vi "action.vi"(0 "HGF_TaskDFSM":refnum<class "HGF_TaskDFSM.lvclass">, 5 "error in (no error)":errorcluster, 8 "HGF_ThreadWorker":refnum<class "HGF_ThreadWorker.lvclass">) -> (10 "dup HGF_ThreadWorker":refnum<class "HGF_ThreadWorker.lvclass">, 14 "dup HGF_TaskDFSM":refnum<class "HGF_TaskDFSM.lvclass">, 19 "error out":errorcluster)   [LabVIEW 2012, in "HGF_DeviceFSM.lvlib" / "HGF_TaskDFSM.lvclass"]
uses:
  HGF_TaskDFSM.lvclass
  HGF_DeviceBaseClasses/HGF_DeviceVisitor/HGF_DeviceVisitor.lvclass
  HGF_DeviceFSM/HGF_DeviceFSM.lvsc/Trigger.ctl
  HGF_DeviceFSM/HGF_DeviceFSM.lvsc
  <vilib>/Statechart/Nodes/EventFiring/NI_SC_EventFiringNode.xnode
  HGF_DeviceFSM/HGF_DeviceFSM.lvsc/Inputs.ctl
  HGF_DeviceFSM/HGF_DeviceFSM.lvsc/Outputs.ctl
  HGF_DeviceFSM/HGF_DeviceFSM.lvsc/State.ctl
  HGF_DeviceFSM/HGF_DeviceFSM.lvsc/StatechartState.ctl
  <vilib>/Statechart/Infrastructure/RTStatechart/RunTime SCN.xnode
  HGF_BaseClasses/HGF_ThreadTask/HGF_ThreadTask.lvclass
  HGF_BaseClasses/HGF_Stop/HGF_Stop.lvclass
  HGF_BaseClasses/HGF_Exception/HGF_Exception.lvclass
  HGF_BaseClasses/HGF_Visitor/HGF_Visitor.lvclass
  HGF_BaseClasses/HGF_Event/HGF_Event.lvclass
  HGF_BaseClasses/HGF_TriggeredEvent/HGF_TriggeredEvent.lvclass
  HGF_BaseClasses/HGF_PVPublisher/HGF_PVPublisher.lvclass
  HGF_DFSMVisitor/HGF_DFSMVisitor.lvclass
  HGF_BaseClasses/HGF_Factory/HGF_Factory.lvclass
  HGF_BaseClasses/HGF_VariantDataObject/HGF_VariantDataObject.lvclass
  HGF_DeviceFSM/HGF_DeviceFSM_Internals.ctl
  HGF_DeviceBaseClasses/HGF_DeviceBaseClasses.lvlib
  <vilib>/Statechart/Common/IntGuid.ctl
  <vilib>/Statechart/Common/NI_SC_LVSCCommonFiles.lvlib
  HGF_DeviceFSM/HGF_DeviceFSM.lvsc/CompanionDiagram.vi/28/SC Main.vi
  <vilib>/Statechart/Common/DbgID.ctl
  HGF_BaseClasses/HGF_ThreadWorker/HGF_ThreadWorker.lvclass
panel:
  out "className":string
  out "Active States":T1
  out "DFSM Internals":T3
  out "SC Loop":i32
  out "Trigger timed out?":bool
  in  "Inputs":T4
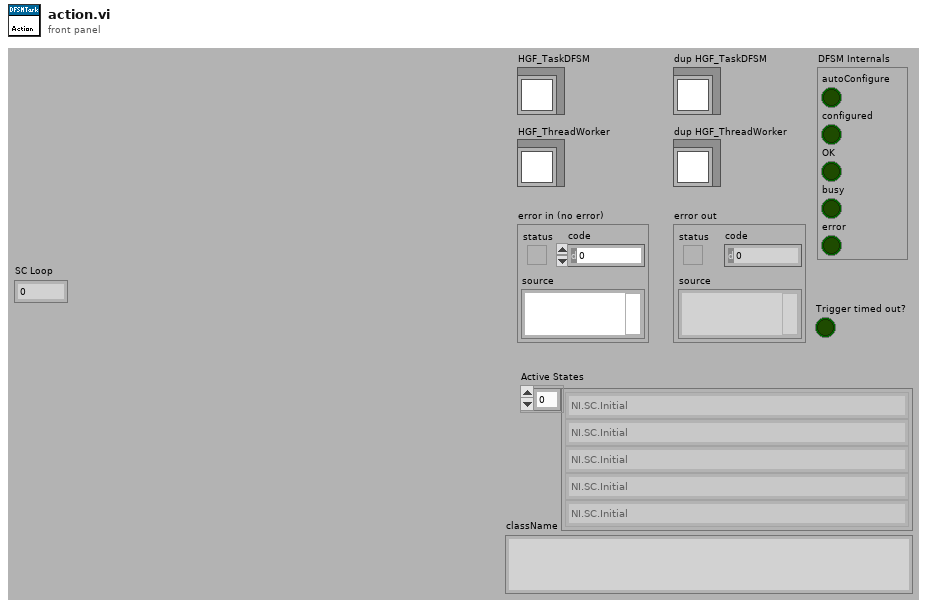
[diagram p1: front panel]
types:
  T1 = typedef "HGF_DeviceFSM.lvlib/HGF_DeviceFSM.lvsc/StatechartState.ctl" = T2[]
  T2 = typedef "HGF_DeviceFSM.lvlib/HGF_DeviceFSM.lvsc/State.ctl" = enum16{"NI.SC.Initial", "NI.SC.History", "NI.SC.ShallowHistory", "NI.SC.Terminal", "Alive", "Alive\\LiveCycle\\Configure", "Alive\\LiveCycle\\Configured", "Alive\\LiveCycle\\Error", "Alive\\LiveCycle\\NotConfigured", "Alive\\LiveCycle\\Configured\\ConfiguredRegion\\Busy", "Alive\\LiveCycle\\Configured\\ConfiguredRegion\\Idle", "Alive\\LiveCycle\\Configured\\ConfiguredRegion\\Idle\\IdleRegion\\Fault", "Alive\\LiveCycle\\Configured\\ConfiguredRegion\\Idle\\IdleRegion\\OK"}
  T3 = typedef "HGF_DeviceBaseClasses.lvlib/HGF_DeviceFSM_Internals.ctl" = cluster{"autoConfigure":bool, "configured":bool, "OK":bool, "busy":bool, "error":bool}
  T4 = typedef "HGF_DeviceFSM.lvlib/HGF_DeviceFSM.lvsc/Inputs.ctl" = cluster{"HGF_DeviceVisitor":refnum<class "HGF_DeviceVisitor.lvclass">, "autoConfigure":bool, "HGF_Factory":refnum<class "HGF_Factory.lvclass">, "DeviceInitData":refnum<class "HGF_VariantDataObject.lvclass">}
  T5 = typedef "HGF_DeviceFSM.lvlib/HGF_DeviceFSM.lvsc/Trigger.ctl" = enum16{"NULL", "configure", "fault", "error", "resetError", "STOP", "visit", "not_configured", "done", "ok", "previsit", "configured"}
  T6 = typedef "NI_SC_LVSCCommonFiles.lvlib/IntGuid.ctl" = cluster{"Data1":u32, "Data2":u16, "Data3":u16, "Data4":u8, "Data5":u8, "Data6":u8, "Data11":u8, "Data9":u8, "Data10":u8, "Data8":u8, "Data7":u8}
  T7 = typedef "NI_SC_LVSCCommonFiles.lvlib/DbgID.ctl" = cluster{"VIRef":u32, "IntGUID":T6}
  T8 = typedef "HGF_DeviceFSM.lvlib/HGF_DeviceFSM.lvsc/Outputs.ctl" = cluster{"HGF_DeviceVisitor":refnum<class "HGF_DeviceVisitor.lvclass">, "DFSM Internals":T3, "error out":errorcluster}
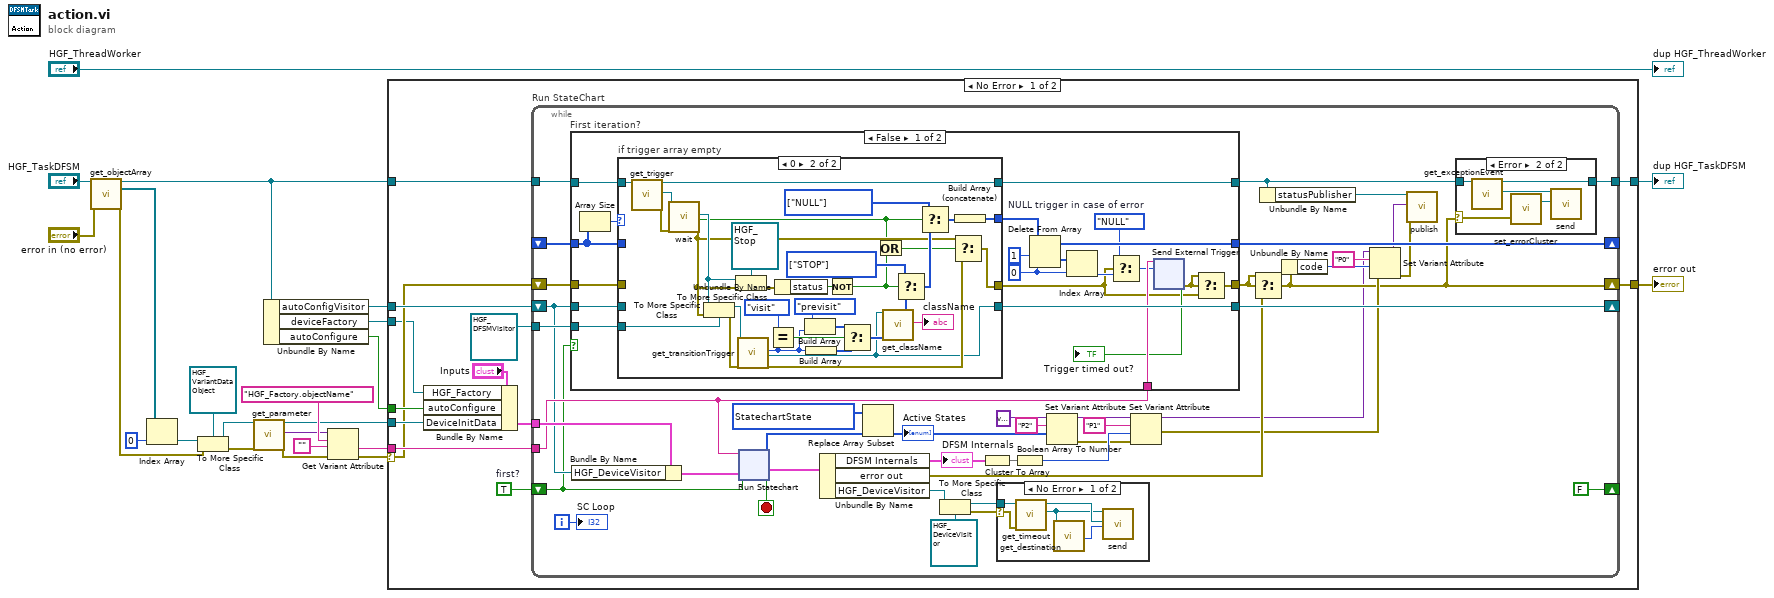
[diagram p0: block diagram]
diagram:
  n1 = call "get_objectArray.vi"("HGF_ThreadTask"="HGF_TaskDFSM", "error in (no error)"="error in (no error)") -> ("dup HGF_ThreadTask"=w17:refnum<class "HGF_TaskDFSM.lvclass">, "objectArray"=w16:refnum<class>[], "error out"=w1:errorcluster)  [unwired: 15 out]
  n2 = Index Array(array=w16, index=0) -> (element=w13:refnum<class>)
  n3 = To More Specific Class(target class=refnum<class "HGF_VariantDataObject.lvclass"> refnum ("HGF_BaseClasses.lvlib:HGF_VariantDataObject.lvclass"), reference=w13, error in=w1) -> (specific class reference=w7:refnum<class "HGF_VariantDataObject.lvclass">, error out=w4:errorcluster)
  n4 = call "get_parameter.vi"("HGF_VariantDataObject"=w7, "error in (no error)"=w4) -> ("dup HGF_VariantDataObject"=w3:refnum<class "HGF_VariantDataObject.lvclass">, "parameter"=w5:variant, "error out"=w6:errorcluster)  [unwired: 15 out]
  n5 = Unbundle By Name(w17) -> ("autoConfigVisitor"=w21:refnum<class "HGF_DeviceVisitor.lvclass">, "deviceFactory"=w2:refnum<class "HGF_Factory.lvclass">, "autoConfigure"=w22:bool)
  n6 = Get Variant Attribute(Variant=w5, name="HGF_Factory.objectName", default value (empty Variant)="", error in=w6) -> (value=w10:string, error out=w9:errorcluster)  [unwired: 2 out]
  n7 = case shown="No Error" w9 {
    selector: w9 -> [w25 w260]
    tunnel: w3 -> [w26 _]
    tunnel: w10 -> [w33 _]
    tunnel: w21 -> [w32 _]
    tunnel: w22 -> [w31 _]
    tunnel: [w28 w260] -> w20
    tunnel: w17 -> [w30 w261]
    tunnel: [w27 w261] -> w19
    tunnel: w2 -> [w24 _]
    frame No Error {
      w36 = TRUE  # first?
      n8 = Bundle By Name(cluster="Inputs", "HGF_Factory"=w24, "autoConfigure"=w31, "DeviceInitData"=w26) -> (w34:T4)
      n9 = while "Run StateChart" {
        tunnel: w33 -> [w66]
        shift-right: [FALSE] -> _
        shift-left: w36 -> [w62]
        tunnel: refnum<class "HGF_DFSMVisitor.lvclass"> refnum ("HGF_DFSMVisitor") -> [w71]
        tunnel: w34 -> [w70]
        shift-right: [w68] -> _
        shift-left: w32 -> [w63]
        shift-right: [w67] -> _
        shift-left: _ -> [w65]
        shift-right: [w46] -> w28
        shift-left: w25 -> [w64]
        tunnel: w30 -> [w58]
        tunnel: [w57] -> w27
        i -> [w75]
        stop <- w39 stop-if-true
        w37 = T1 [enum."NI.SC.Initial", enum."NI.SC.Initial", enum."NI.SC.Initial", enum."NI.SC.Initial", enum."NI.SC.Initial", enum."NI.SC.Initial"] items=["NI.SC.Initial", "NI.SC.History", "NI.SC.ShallowHistory", "NI.SC.Terminal", "Alive", "Alive\\LiveCycle\\Configure", "Alive\\LiveCycle\\Configured", "Alive\\LiveCycle\\Error", "Alive\\LiveCycle\\NotConfigured", "Alive\\LiveCycle\\Configured\\ConfiguredRegion\\Busy", "Alive\\LiveCycle\\Configured\\ConfiguredRegion\\Idle", "Alive\\LiveCycle\\Configured\\ConfiguredRegion\\Idle\\IdleRegion\\Fault", "Alive\\LiveCycle\\Configured\\ConfiguredRegion\\Idle\\IdleRegion\\OK"] ("Active States")
        n10 = case "First iteration?" shown="False" w62 {
          tunnel: w71 -> [w104 _]
          tunnel: [w103 w157] -> w68
          tunnel: [w102 w159] -> w67
          tunnel: w66 -> [w97 _]
          tunnel: w65 -> [w96 w159]
          tunnel: [w84 w158] -> w60
          tunnel: w64 -> [w95 w158]
          tunnel: w63 -> [w93 w157]
          tunnel: w58 -> [w91 w156]
          tunnel: [w90 w156] -> w56
          frame False {
            w87 = Trigger."NULL"  # NULL trigger in case of error
            w98 = 0 ("index")
            n11 = Array Size(array=w96) -> (size(s)=w92:i32)
            n12 = case "if trigger array empty" shown="0" w92 {
              tunnel: w104 -> [_ w128]
              tunnel: [w106 w109] -> w103
              tunnel: [w108 w135] -> w101
              tunnel: [w107 w116] -> w85
              tunnel: w96 -> [w108 _]
              tunnel: w93 -> [w106 _]
              tunnel: w95 -> [w107 _]
              tunnel: w91 -> [w105 w134]
              tunnel: [w105 w133] -> w90
              frame Default {
              }
              frame 0 {
                w127 = T5[] [enum."STOP"] items=["NULL", "configure", "fault", "error", "resetError", "STOP", "visit", "not_configured", "done", "ok", "previsit", "configured"]
                w126 = T5[] [enum."NULL"] items=["NULL", "configure", "fault", "error", "resetError", "STOP", "visit", "not_configured", "done", "ok", "previsit", "configured"]
                n13 = call "get_trigger.vi"("HGF_ThreadTask"=w134) -> ("dup HGF_ThreadTask"=w133:refnum<class "HGF_TaskDFSM.lvclass">, "trigger"=w137:refnum<class "HGF_Event.lvclass">, "error out"=w136:errorcluster)  [unwired: 1 in, 15 out]
                n14 = call-dynamic "wait.vi"("HGF_Event"=w137, "error in (no error)"=w136) -> ("Object"=w139:refnum<class>, "timed out"=w113:bool, "error out"=w115:errorcluster)  [unwired: 2 in, 13 out]
                n15 = To More Specific Class(target class=w128, reference=w139, error in=w115) -> (specific class reference=w111:refnum<class "HGF_DFSMVisitor.lvclass">, error out=w125:errorcluster)
                n16 = To More Specific Class(target class=refnum<class "HGF_Stop.lvclass"> refnum ("HGF_BaseClasses.lvlib:HGF_Stop.lvclass"), reference=w139, error in=w115) -> (error out=w132:errorcluster)  [unwired: 1 out]
                n17 = call-dynamic "get_transitionTrigger.vi"("HGF_DFSMVisitor"=w111, "error in (no error)"=w125) -> ("Trigger"=w119:T5, "deviceVisitor"=w109:refnum<class "HGF_DeviceVisitor.lvclass">, "error out"=w117:errorcluster)  [unwired: 14 in, 1 out]
                n18 = Equal?(x=Trigger."visit" ("Trigger"), y=w119) -> (x = y?=w120:bool)
                n19 = Unbundle By Name(w132) -> ("status"=w131:bool)
                n20 = Build Array(Trigger."previsit" ("Trigger"), w119) -> (w122:T5[])
                n21 = Build Array(w119) -> (w118:T5[])
                n22 = Not(x=w131) -> (.not. x?=w114:bool)
                n23 = Select(t=w122, s=w120, f=w118) -> (s? t:f=w121:T5[])
                n24 = Or(x=w113, y=w114) -> (x .or. y?=w112:bool)
                n25 = call "get_className.vi"("HGF_Factory"=w109) -> ("className"=→"className":string)  [unwired: 1 in, 17 out]
                n26 = Select(t=w127, s=w114, f=w121) -> (s? t:f=w129:T5[])
                n27 = Select(t=w126, s=w113, f=w129) -> (s? t:f=w130:T5[])
                n28 = Select(t=w115, s=w112, f=w117) -> (s? t:f=w116:errorcluster)
                n29 = Build Array (concatenate)(w130) -> (w135:T5[])
              }
            }
            n30 = Delete From Array(array=w101, length=1, index=w98) -> (deleted portion=w99:T5[], array with subset deleted=w102:T5[])
            n31 = Index Array(array=w99, index=w98) -> (element=w89:T5)
            n32 = Select(t=w87, s=w85, f=w89) -> (s? t:f=w88:T5)
            n33 = xnode "Send External Trigger"("Instance Name"=w97, "Trigger"=w88) -> ("Timed out?"=→"Trigger timed out?":bool, "error out"=w86:errorcluster)  [unwired: 1 in]
            n34 = Select(t=w86, s=w86, f=w85) -> (s? t:f=w84:errorcluster)
          }
          frame True {
          }
        }
        n35 = Bundle By Name(cluster=w70, "HGF_DeviceVisitor"=w63) -> (w69:T4)
        n36 = xnode "Run Statechart"("Init?"=w62, "Inputs"=w69, "Instance Name"=w66) -> ("Terminated?"=w39:bool, "Outputs"=w76:T8, "Active States"=w38:T1)
        "Active States" <- w38
        n37 = Unbundle By Name(w76) -> ("DFSM Internals"=w54:T3, "error out"=w61:errorcluster, "HGF_DeviceVisitor"=w74:refnum<class "HGF_DeviceVisitor.lvclass">)
        "DFSM Internals" <- w54
        n38 = Replace Array Subset(array=w37, new element=w38) -> ()  [unwired: 1 in, 1 out]
        n39 = To More Specific Class(target class=refnum<class "HGF_DeviceVisitor.lvclass"> refnum ("HGF_DeviceBaseClasses.lvlib:HGF_DeviceVisitor.lvclass"), reference=w74) -> (specific class reference=w73:refnum<class "HGF_DeviceVisitor.lvclass">, error out=w72:errorcluster)  [unwired: 1 in]
        n40 = Cluster To Array(cluster=w54) -> (array=w53:bool[])
        n41 = case shown="No Error" w72 {
          selector: w72 -> [w258 _]
          tunnel: w73 -> [w259 _]
          frame No Error {
            n42 = call "get_destination.vi"("error in (no error)"=w258, "HGF_Visitor"=w259) -> ("destination"=w256:refnum<class "HGF_TriggeredEvent.lvclass">, "dup HGF_Visitor"=w257:refnum<class "HGF_DeviceVisitor.lvclass">)  [unwired: 8 out]
            n43 = call "get_timeout.vi"("HGF_Event.lvclass in"=w256) -> ("timeout"=w255:i32)  [unwired: 1 in, 17 out]
            n44 = call-dynamic "send.vi"("HGF_Event"=w256, "Object"=w257, "timeout in ms (-1)"=w255) -> ()  [unwired: 2 in, 15 out]
          }
          frame Error {
          }
        }
        n45 = Boolean Array To Number(Boolean array=w53) -> (number=w52:u32)
        n46 = Set Variant Attribute(Variant=variant ("variant"), name="P2", value=w38) -> (Variant out=w41:variant, error out=w40:errorcluster)  [unwired: 1 in, 1 out]
        n47 = Set Variant Attribute(Variant=w41, name="P1", value=w52, error in=w40) -> (Variant out=w44:variant, error out=w49:errorcluster)  [unwired: 1 out]
        n48 = Select(t=w60, s=w60, f=w61) -> (s? t:f=w46:errorcluster)
        n49 = Unbundle By Name(w56) -> ("statusPublisher"=w55:refnum<class "HGF_PVPublisher.lvclass">)
        n50 = Unbundle By Name(w46) -> ("code"=w45:i32)
        n51 = Set Variant Attribute(Variant=w44, name="P0", value=w45, error in=w49) -> (Variant out=w47:variant, error out=w48:errorcluster)  [unwired: 1 out]
        n52 = call-dynamic "publish.vi"("HGF_PVPublisher"=w55, "data"=w47, "error in (no error)"=w48) -> ()  [unwired: 2 in, 15 out]
        n53 = case shown="Error" w46 {
          selector: w46 -> [_ w79]
          tunnel: w56 -> [w78 w81]
          tunnel: [w78 w80] -> w57
          frame No Error {
          }
          frame Error {
            n54 = call "get_exceptionEvent.vi"("HGF_ThreadTask"=w81) -> ("dup HGF_ThreadTask"=w80:refnum<class "HGF_TaskDFSM.lvclass">, "exceptionEvent"=w82:refnum<class "HGF_Event.lvclass">)  [unwired: 1 in, 16 out]
            n55 = call "set_errorCluster.vi"("error in (no error)"=w79) -> ("dup HGF_Exception"=w83:refnum<class "HGF_Exception.lvclass">)  [unwired: 1 in]
            n56 = call-dynamic "send.vi"("HGF_Event"=w82, "Object"=w83) -> ()  [unwired: 3 in, 15 out]
          }
        }
        "SC Loop" <- w75
      }
    }
    frame Error {
    }
  }
  "error out" <- w20
  "dup HGF_TaskDFSM" <- w19
  "dup HGF_ThreadWorker" <- "HGF_ThreadWorker"
